vi "solar_voy TCP Listener Create.vi"(7 "Instance in":i32, 8 "error in (no error)":errorcluster, 10 "Port":u16, 11 "Voyager Refnum in":T1) -> (0 "error out":errorcluster, 2 "Listener ID":refnum<k5>, 3 "Voyager Refnum out":T1)   [LabVIEW 2018]
doc: "This creates a TCP listener."
uses:
  solar_voy_ctl Voyager Refnum.ctl
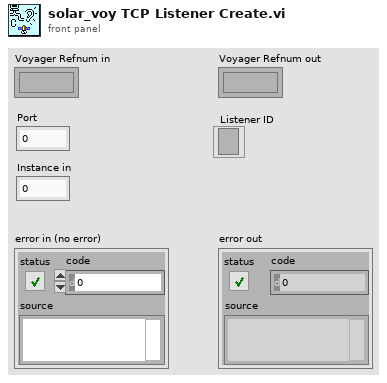
[diagram p1: front panel]
types:
  T1 = typedef "solar_voy_ctl Voyager Refnum.ctl" = refnum<k1>
  T2 = typedef "solar_voy_ctl Voyager.ctl" = cluster{"PACKETS":T3[], "COSMOS_Root":path, "CMD_HDR":T8, "TLM_HDR":T8, "TCPs":T9[], "VoyagerIDOffset":cluster{"VoyagerIDOffset":u16[], "Target Names":string[]}}
  T3 = typedef "solar_voy_def_ctl PACKET.ctl" = cluster{"PACKET_ID":T4, "ENDIAN":enum8{"BIG", "LITTLE"}, "DESC":string, "HZRD":bool, "ITEMS":T5[], "NoExport":bool, "last_time":timestamp, "last_count":u32, "last_data":string}
  T4 = typedef "solar_voy_def_ctl PACKET_ID.ctl" = cluster{"ID":u16, "CMD":enum8{"CMD", "TLM"}, "TARGET":string, "PACKET":string}
  T5 = typedef "solar_voy_def_ctl ITEM.ctl" = cluster{"NAME":string, "OFFSET":i32, "SIZE":i32, "TYPE":T6, "EACH_SIZE":i32, "LVTYPE":T7, "MIN":dbl, "MAX":dbl, "DEFAULT":string, "DESC":string, "ID":bool, "MODIFIERS":variant, "last_value":variant}
  T6 = typedef "solar_voy_def_ctl ITEM TYPE.ctl" = enum8{"BLOCK", "INT", "UINT", "FLOAT", "STRING"}
  T7 = typedef "solar_type Item Type.ctl" = enum16{"NULL", "UNKNOWN", "CLUSTER", "I8", "I16", "I32", "I64", "U8", "U16", "U32", "U64", "U8_ENUM", "U16_ENUM", "U32_ENUM", "SGL", "DBL", "BOOLEAN", "STRING", "PATH", "VISA", "TAG", "TIME", "I8_1D", "I16_1D", "I32_1D", "I64_1D", "U8_1D", "U16_1D", "U32_1D", "U64_1D", "U8_ENUM_1D", "U16_ENUM_1D", "U32_ENUM_1D", "SGL_1D", "DBL_1D", "BOOLEAN_1D", "STRING_1D", "PATH_1D", "VISA_1D", "TAG_1D", "TIME_1D", "I8_2D", "I16_2D", "I32_2D", "I64_2D", "U8_2D", "U16_2D", "U32_2D", "U64_2D", "U8_ENUM_2D", "U16_ENUM_2D", "U32_ENUM_2D", "SGL_2D", "DBL_2D", "BOOLEAN_2D", "STRING_2D", "PATH_2D", "VISA_2D", "TAG_2D", "TIME_2D"}
  T8 = typedef "solar_voy_def_ctl HDR.ctl" = cluster{"ITEMS":T5[], "LENGTH_NAME":string, "LENGTH_VALUE_OFFSET":i32, "ID_NAME":string, "ENDIAN":enum8{"BIG", "LITTLE"}, "GUID_NAME":string, "DEFAULT_TARGET":string, "DEFAULT_PACKET":string, "DEFAULT_ERROR":string}
  T9 = typedef "solar_voy_ctl TCP.ctl" = cluster{"Connected":bool, "Port":u16, "Listener":refnum<k5>, "ServerIP":string, "TCP":refnum<k5>, "Setup":T10, "VIRefnum":refnum<vi>, "TARGETS_CMD":string[], "TARGETS_TLM":string[]}
  T10 = typedef "solar_voy_ctl Port Setup.ctl" = enum8{"SERVER", "CLIENT", "SERVER_CMD", "SERVER_TLM"}
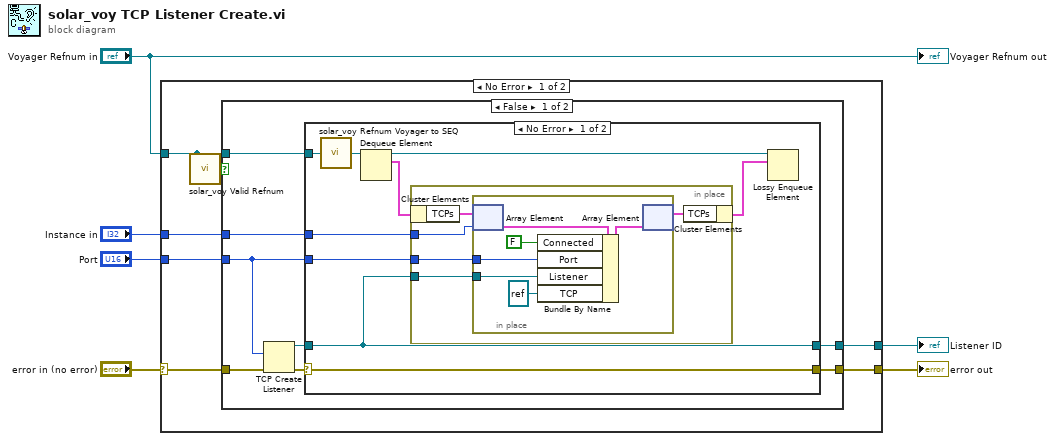
[diagram p0: block diagram]
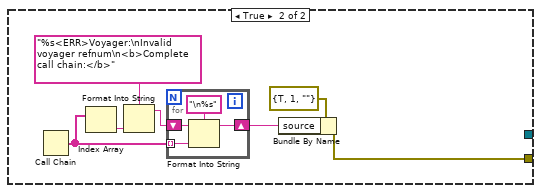
[diagram p3: hidden frame]
diagram:
  n1 = case shown="No Error" "error in (no error)" {
    selector: "error in (no error)" -> [w9 w54]
    tunnel: [w13 _] -> w6
    tunnel: "Port" -> [w12 _]
    tunnel: "Voyager Refnum in" -> [w8 _]
    tunnel: "Instance in" -> [w11 _]
    tunnel: [w10 w54] -> w2
    frame No Error {
      n2 = call "solar_voy Valid Refnum.vi"("Voyager Refnum"=w8) -> ("Invalid Refnum?"=w7:bool)
      n3 = case shown="False" w7 {
        tunnel: [w21 _] -> w13
        tunnel: w12 -> [w18 _]
        tunnel: w11 -> [w17 _]
        tunnel: [w16 w44] -> w10
        tunnel: w9 -> [w15 _]
        tunnel: w8 -> [w14 _]
        frame False {
          n4 = TCP Create Listener(8:w15, 10:w18) -> (0:w20:errorcluster, 3:w19:refnum<k5>)  [unwired: 4 out]
          n5 = case shown="No Error" w20 {
            selector: w20 -> [w25 w42]
            tunnel: w14 -> [w24 _]
            tunnel: w18 -> [w28 _]
            tunnel: w17 -> [w27 _]
            tunnel: w19 -> [w26 _]
            tunnel: [w26 _] -> w21
            tunnel: [w25 w42] -> w16
            frame No Error {
              n6 = call "solar_voy Refnum Voyager to SEQ.vi"("Voyager Refnum"=w24) -> ("Voyager SEQ"=w30:refnum<queue>)
              n7 = Dequeue Element(queue=w30) -> (queue out=w29:refnum<queue>, element=w23:T2)  [unwired: 2 in, 2 out]
              n8 = in-place {
                in-place-border: w28 -> [w35]
                in-place-border: w27 -> [w34]
                in-place-border: w26 -> [w33]
                n9 = in-place-cluster #1(w23) -> ("TCPs"=w32:T9[])
                n10 = in-place {
                  in-place-border: w35 -> [w38]
                  in-place-border: w33 -> [w37]
                  n11 = in-place-array #2(w32, w34) -> (w41:T9)
                  n12 = Bundle By Name(cluster=w41, "Connected"=FALSE, "Port"=w38, "Listener"=w37, "TCP"=refnum<k5> refnum) -> (w40:T9)
                  n13 = in-place-array #2(w40) -> (w31:T9[])  [unwired: 1 out]
                }
                n14 = in-place-cluster #1("TCPs"=w31) -> (w22:T2)
              }
              n15 = Lossy Enqueue Element(queue=w29, element=w22) -> ()  [unwired: 1 in, 4 out]
            }
            frame Error {
            }
          }
        }
        frame True {
          n16 = Call Chain() -> (call chain=w45:string[])
          n17 = Index Array(array=w45) -> (element=w47:string)  [unwired: 1 in]
          n18 = Format Into String(format string="%s<ERR>Voyager:\nInvalid voyager refnum\n<b>Complete call chain:</b>", w47) -> (resulting string=w46:string)  [unwired: 2 in, 1 out]
          n19 = for {
            tunnel: w45 -> [w53] mode=indexing
            shift-right: [w52] -> w43
            shift-left: w46 -> [w51]
            n20 = Format Into String(format string="\n%s", initial string=w51, w53) -> (resulting string=w52:string)  [unwired: 1 in, 1 out]
          }
          n21 = Bundle By Name(cluster=errorcluster {"status"=TRUE, "code"=1, "source"=""} ("Error"), "source"=w43) -> (w44:errorcluster)
        }
      }
    }
    frame Error {
    }
  }
  "Listener ID" <- w6
  "error out" <- w2
  "Voyager Refnum out" <- "Voyager Refnum in"
